vi "Send CCD Status.vi"(8 "error in (no error)":errorcluster, 11 "Stream in":refnum<class "Stream.lvclass">) -> (0 "error out":errorcluster, 3 "Stream out":refnum<class "Stream.lvclass">)   [LabVIEW 2018, in "Stream.lvclass"]
uses:
  Stream.lvclass
  Stream.lvclass/Stream.ctl
  Interface/Interface.lvclass
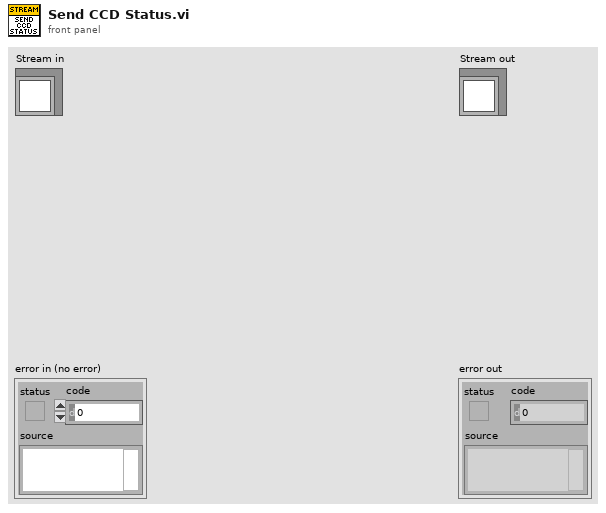
[diagram p1: front panel]
types:
  T1 = cluster{"CUBE_EXPOSURE_TIME":sgl, "CUBES_DONE":u16, "LAST_IMAGE_NAME":string, "DISK_SPACE":u16, "FRAMES_DONE":u16, "CCD_STATUS":string, "CURRENT_TEMPERATURE":i16, "TEMPERATURE_STATUS":string, "FRAME_EXPOSURE_TIME":u16}
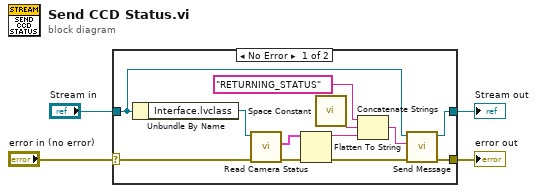
[diagram p0: block diagram]
diagram:
  n1 = case shown="No Error" "error in (no error)" {
    selector: "error in (no error)" -> [w11 w18]
    tunnel: [w16 w18] -> w3
    tunnel: [w14 w17] -> w1
    tunnel: "Stream in" -> [w15 w17]
    frame No Error {
      n2 = Unbundle By Name(w15) -> ("Interface.lvclass"=w12:refnum<class "Interface.lvclass">)
      n3 = call "Read Camera Status.vi"("error in (no error)"=w11, "Interface in"=w12) -> ("error out"=w10:errorcluster, "Camera Status"=w13:T1)  [unwired: 7 in, 1 out]
      n4 = Flatten To String(anything=w13, error in (no error)=w10) -> (data string=w6:string, error out=w9:errorcluster)  [unwired: 2 in, 1 out]
      n5 = call <vilib>:"Space Constant.vi"() -> ("String"=w7:string)
      n6 = Concatenate Strings("RETURNING_STATUS", w7, w6) -> (w5:string)
      n7 = call "Send Message.vi"("error in (no error)"=w9, "Message"=w5, "Stream in"=w15) -> ("error out"=w16:errorcluster, "Stream out"=w14:refnum<class "Stream.lvclass">)  [unwired: 7 in]
    }
    frame Error {
    }
  }
  "error out" <- w3
  "Stream out" <- w1
